vi "Calibrate ADC.vi"(8 "error in (no error)":errorcluster, 11 "VISA resource name":refnum<visa-resource-name>) -> (0 "error out":errorcluster, 2 "Calibration Result":bool, 3 "VISA resource name out":refnum<visa-resource-name>)   [LabVIEW 2013, in "Agilent 3446X Series.lvlib"]
doc: "Performs a low-level calibration of the ADC (analog-to-digital converter) circuitry.\n\n<b>Note(s):</b>\nThis vi is not supported for EDU34450A model."
uses:
  <instrlib>/Agilent 3446X Series/Agilent 3446X Series.lvlib
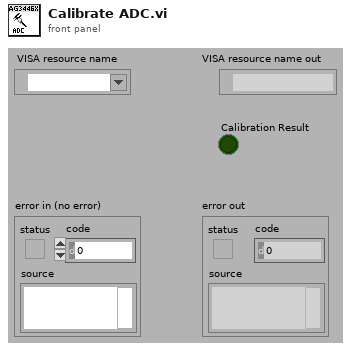
[diagram p1: front panel]
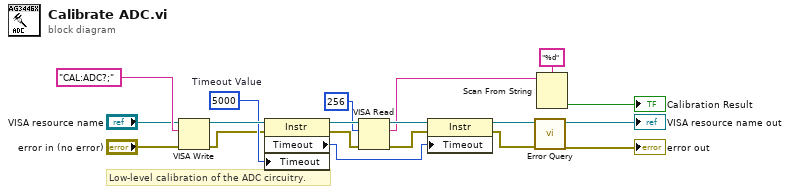
[diagram p0: block diagram]
diagram:
  w13 = u32 5000  # Timeout Value
  # "Low-level calibration of the ADC circuitry."
  n1 = VISA Write(VISA resource name="VISA resource name", write buffer="CAL:ADC?;", error in (no error)="error in (no error)") -> (VISA resource name out=w14:refnum<visa-resource-name>, error out=w11:errorcluster)  [unwired: 1 out]
  n2 = property class="Instr"(reference=w14, error in=w11, "Timeout"=w13) -> (reference out=w12:refnum<visa-resource-name>, error out=w10:errorcluster, "Timeout"=w6:u32)
  n3 = VISA Read(VISA resource name=w12, byte count=u32 256, error in (no error)=w10) -> (VISA resource name out=w8:refnum<visa-resource-name>, read buffer=w2:string, error out=w7:errorcluster)  [unwired: 1 out]
  n4 = property class="Instr"(reference=w8, error in=w7, "Timeout"=w6) -> (reference out=w5:refnum<visa-resource-name>, error out=w4:errorcluster)
  n5 = call <instrlib>:"Error Query.vi"("error in (no error)"=w4, "VISA resource name"=w5) -> ("error out"=→"error out":errorcluster, "VISA resource name out"=→"VISA resource name out":refnum<visa-resource-name>)  [unwired: 8 out]
  n6 = Scan From String(format string="%d", input string=w2) -> (output 1=→"Calibration Result":bool)  [unwired: 2 in, 4 out]
